vi "Config.vi"(8 "error in (no error)":errorcluster, 11 "MSX-E3711 in":refnum<class "MSX-E3711.lvclass">) -> (0 "error out":errorcluster, 2 "HAL Config Data":T1, 3 "MSX-E3711 out":refnum<class "MSX-E3711.lvclass">)   [LabVIEW 2014, in "MSX-E3711.lvlib" / "MSX-E3711.lvclass"]
uses:
  MSX-E3711.lvclass
  DriverMasterSync/build/DriverMasterSync.lvlibp/Modules/HAL/TypeDefs/HAL Config Data.ctl
  DriverMasterSync/build/DriverMasterSync.lvlibp/Modules/HAL/DriverMasterSync/DriverMasterSyncClass/DriverMasterSync.lvclass
  DriverMasterSync/build/DriverMasterSync.lvlibp
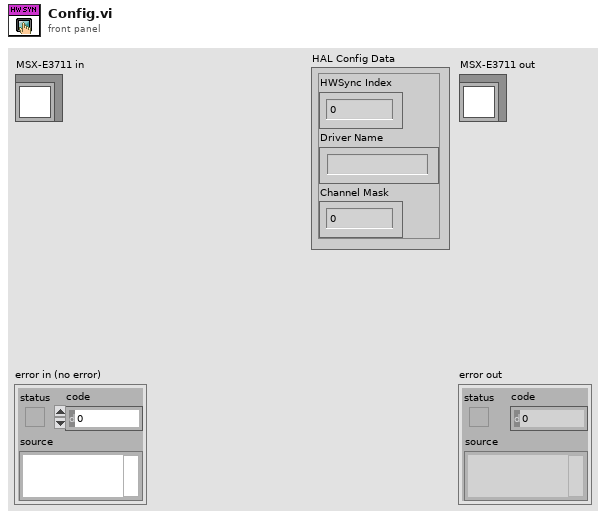
[diagram p1: front panel]
types:
  T1 = typedef "DriverMasterSync.lvlibp/HAL Config Data.ctl" = cluster{"HWSync Index":u32, "Driver Name":string, "Channel Mask":u64}
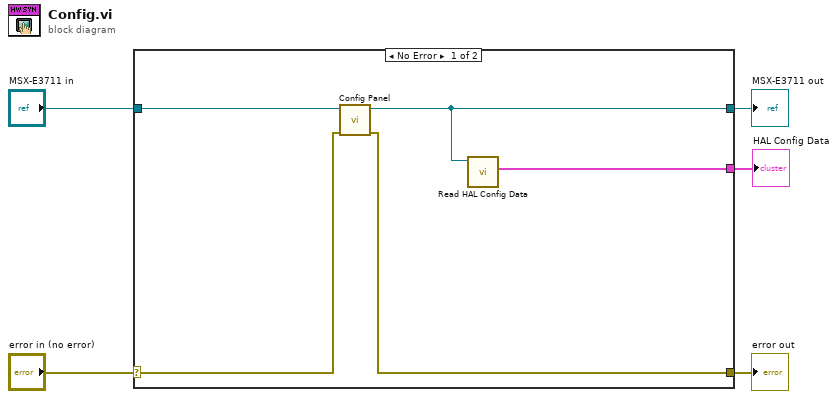
[diagram p0: block diagram]
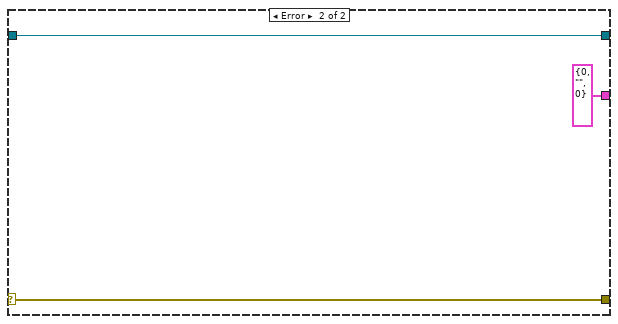
[diagram p2: hidden frame]
diagram:
  n1 = case shown="No Error" "error in (no error)" {
    selector: "error in (no error)" -> [w7 w13]
    tunnel: [w6 w13] -> w4
    tunnel: [w9 w12] -> w2
    tunnel: "MSX-E3711 in" -> [w10 w12]
    tunnel: [w8 T1 {"HWSync Index"=0, "Driver Name"="", "Channel Mask"=0} ("HAL Config Data")] -> w1
    frame No Error {
      n2 = call "Config Panel.vi"("Error In"=w7, "MSX-E3711 in"=w10) -> ("Error Out"=w6:errorcluster, "MSX-E3711 out"=w9:refnum<class "MSX-E3711.lvclass">)  [unwired: 7 in]
      n3 = call "Read HAL Config Data.vi"("DriverMasterSync in"=w9) -> ("HAL Config Data"=w8:T1)  [unwired: 8 in, 2 out]
    }
    frame Error {
    }
  }
  "error out" <- w4
  "MSX-E3711 out" <- w2
  "HAL Config Data" <- w1
